vi "First Matched Config File_lvcicd.vi"(6 "pattern(ini by default)":string="*.ini", 8 "Recrusively(F)":bool, 11 "Searching Directory":path) -> (3 "Matched Config File":path)   [LabVIEW 2014, in "_lvcicd_support_2014.lvlib"]
uses:
  <userlib>/_OpenG.lib/file/file.llb/Build Path - File Names Array__ogtk.vi
  _lvcicd_support_2014.lvlib
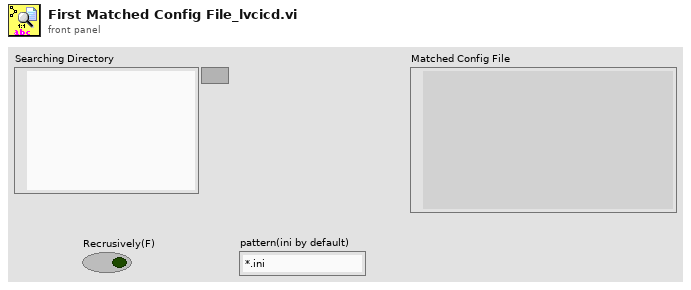
[diagram p1: front panel]
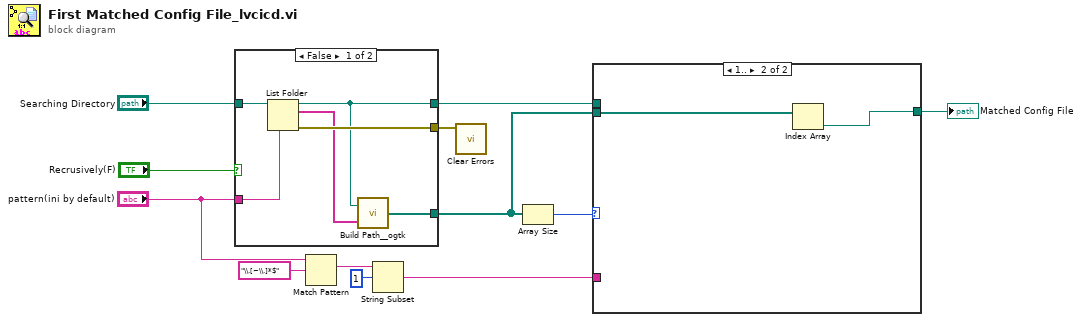
[diagram p0: block diagram]
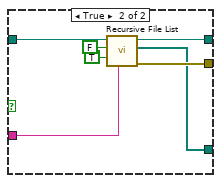
[diagram p2: hidden frame]
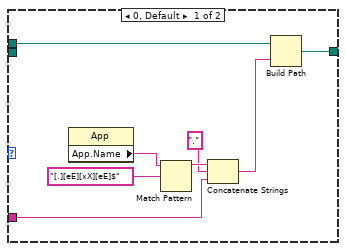
[diagram p3: hidden frame]
diagram:
  n1 = case shown="False" "Recrusively(F)" {
    tunnel: [w18 w23] -> w12
    tunnel: "pattern(ini by default)" -> [w16 w21]
    tunnel: "Searching Directory" -> [w15 w24]
    tunnel: [w14 w22] -> w9
    tunnel: [w13 w25] -> w8
    frame False {
      n2 = List Folder(path=w15, pattern=w16) -> (path out=w13:path, filenames=w17:string[], error out=w18:errorcluster)  [unwired: 2 in, 1 out]
      n3 = call-poly <userlib>:"Build Path__ogtk.vi"("name or relative path"=w17, "base path"=w13) -> ("appended path"=w14:path[])
    }
    frame True {
      n4 = call <vilib>:"Recursive File List.vi"("pattern"=w21, "Continue Recursing on Error? (F)"=TRUE, "Treat LLBs as Folders?"=FALSE, "Folder Path"=w24) -> ("error out"=w23:errorcluster, "All Files in Dir"=w22:path[], "dup Folder Path"=w25:path)  [unwired: 3 in, 2 out]
    }
  }
  n5 = Match Pattern(string="pattern(ini by default)", regular expression="\\.[~\\.]*$") -> (match substring=w6:string)  [unwired: 4 out]
  n6 = String Subset(string=w6, offset (0)=1) -> (substring=w2:string)  [unwired: 1 out]
  n7 = call <vilib>:"Clear Errors.vi"("error in (no error)"=w12) -> ()  [unwired: 5 in, 2 out]
  n8 = Array Size(array=w9) -> (size(s)=w10:i32)
  n9 = case shown="1.." w10 {
    tunnel: w9 -> [_ w35]
    tunnel: w8 -> [w33 _]
    tunnel: [w32 w34] -> w11
    tunnel: w2 -> [w26 _]
    frame 0, Default {
      n10 = property class="App"() -> ("App.Name"=w31:string)  [unwired: 2 in, 2 out]
      n11 = Match Pattern(string=w31, regular expression="[.][eE][xX][eE]$") -> (before substring=w29:string)  [unwired: 1 in, 3 out]
      n12 = Concatenate Strings(w29, "." ("string"), w26) -> (w28:string)
      n13 = Build Path(base path=w33, name or relative path=w28) -> (appended path=w32:path)
    }
    frame 1.. {
      n14 = Index Array(array=w35) -> (element=w34:path)  [unwired: 1 in]
    }
  }
  "Matched Config File" <- w11
